vi "RenameEventFile.vi"(8 "error in (no error)":errorcluster, 10 "New File Name (with extension)":string, 11 "object in":refnum<class "EventLogger_Actor.lvclass">) -> (0 "error out":errorcluster, 3 "object out":refnum<class "EventLogger_Actor.lvclass">)   [LabVIEW 2014, in "EventLogger_Actor.lvlib" / "EventLogger_Actor.lvclass"]
uses:
  EventLogger_Actor.lvclass
  EventLogger_Actor.lvclass/EventLogger_Actor.ctl
  <userlib>/_OpenG.lib/file/file.llb/Strip Path - Traditional__ogtk.vi
  <userlib>/_OpenG.lib/file/file.llb/Build Path - Traditional__ogtk.vi
panel:
  # "BSD 2-Clause License\n\nCopyright (c) 2018, Ajay www.digiajay.com\nAll rights reserved.\n\nRedistribution and use in source and binary forms, with or without\nmodification, are permitted provided that the following conditions are met:\n\n* Redistributions of source code must retain the above copyright notice, this\n  list of conditions and the following disclaimer.\n\n* Redistributions in binary form must reproduce the above copyright notice,\n  this list of conditions and the following disclaimer in the documentation\n  and/or other materials provided with the distribution.\n\nTHIS SOFTWARE IS PROVIDED BY THE COPYRIGHT HOLDERS AND CONTRIBUTORS \"AS IS\"\nAND ANY EXPRESS OR IMPLIED WARRANTIES, INCLUDING, BUT NOT LIMITED TO, THE\nIMPLIED WARRANTIES OF MERCHANTABILITY AND FITNESS FOR A PARTICULAR PURPOSE ARE\nDISCLAIMED. IN NO EVENT SHALL THE COPYRIGHT HOLDER OR CONTRIBUTORS BE LIABLE\nFOR ANY DIRECT, INDIRECT, INCIDENTAL, SPECIAL, EXEMPLARY, OR CONSEQUENTIAL\nDAMAGES (INCLUDING, BUT NOT LIMITED TO, PROCUREMENT OF SUBSTITUTE GOODS OR\nSERVICES; LOSS OF USE, DATA, OR PROFITS; OR BUSINESS INTERRUPTION) HOWEVER\nCAUSED AND ON ANY THEORY OF LIABILITY, WHETHER IN CONTRACT, STRICT LIABILITY,\nOR TORT (INCLUDING NEGLIGENCE OR OTHERWISE) ARISING IN ANY WAY OUT OF THE USE\nOF THIS SOFTWARE, EVEN IF ADVISED OF THE POSSIBILITY OF SUCH DAMAGE."
  # "Connector Pane"
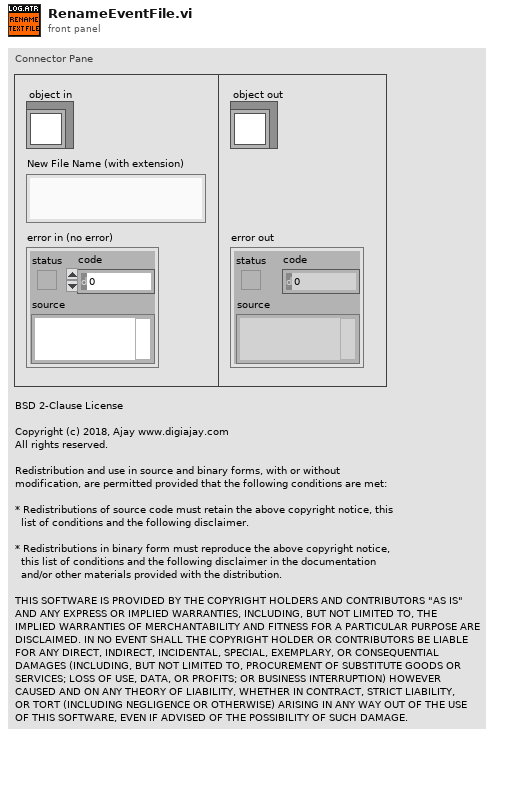
[diagram p1: front panel]
types:
  T1 = enum16{"open", "replace", "create", "open or create", "replace or create", "replace or create with confirmation"}
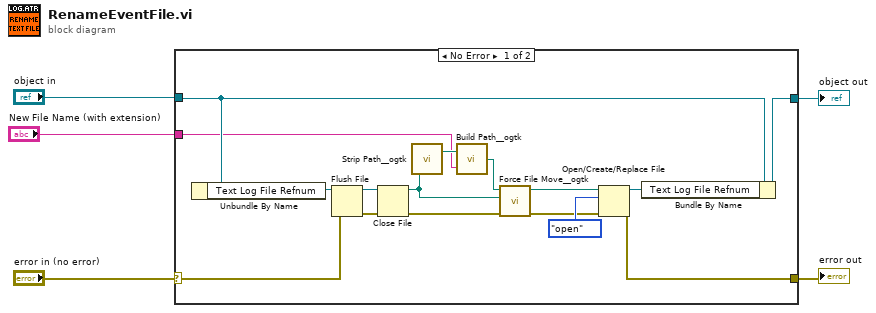
[diagram p0: block diagram]
diagram:
  n1 = case shown="No Error" "error in (no error)" {
    selector: "error in (no error)" -> [w21 w23]
    tunnel: [w9 w23] -> w4
    tunnel: [w19 w22] -> w2
    tunnel: "object in" -> [w20 w22]
    tunnel: "New File Name (with extension)" -> [w8 _]
    frame No Error {
      n2 = Unbundle By Name(w20) -> ("Text Log File Refnum"=w18:refnum<file>)
      n3 = Flush File(refnum=w18, error in=w21) -> (refnum out=w17:refnum<file>, error out=w13:errorcluster)
      n4 = Close File(refnum=w17, error in=w13) -> (path=w7:path, error out=w11:errorcluster)
      n5 = call-poly <userlib>:"Strip Path__ogtk.vi"("path"=w7) -> ("stripped path"=w12:path)  [unwired: 1 out]
      n6 = call-poly <userlib>:"Build Path__ogtk.vi"("name or relative path"=w8, "base path"=w12) -> ("appended path"=w6:path)
      n7 = call <userlib>:"Force File Move__ogtk.vi"("error in (no error)"=w11, "source"=w7, "target"=w6) -> ("error out"=w10:errorcluster, "target out"=w15:path)  [unwired: 3 in]
      n8 = Open/Create/Replace File(file path (use dialog)=w15, error in=w10, operation (0:open)=T1."open") -> (refnum out=w14:refnum<file>, error out=w9:errorcluster)  [unwired: 3 in, 1 out]
      n9 = Bundle By Name(cluster=w20, "Text Log File Refnum"=w14) -> (w19:refnum<class "EventLogger_Actor.lvclass">)
    }
    frame Error {
    }
  }
  "error out" <- w4
  "object out" <- w2
